vi "界面UI.vi"() -> ()   [LabVIEW 2016, in "德润DR803F超标留样.lvlib"]
uses:
  <vilib>/Utility/miscctls.llb/LVPointTypeDef.ctl
  <vilib>/Utility/config.llb/NI_LVConfig.lvlib
panel:
  in  "超标浓度配置":bool
  out "仪器状态":T1 {"门状态" items=["关闭", "打开"]; "采样模式" items=["定时留样"=1, "时间等比"=2, "同步留样"=3, "外控留样"=4, "超标留样"=5]; "工作进程" items=["清洗管路初始化", "采样瓶位置初始化", "采样瓶排空", "清洗管下降", "采样瓶清洗", "清洗管上升", "外置泵延时", "管路润洗", "进样1", "进样2", "排空管路", "采样瓶位置调整", "待机"]; "仪器时间" format="%<%Y/%m/%d %H:%M:%S>T"; "工作状态" items=["停止", "运行"]}
  in  "采样瓶排空":bool
  out "超标留样等待时间/s":dbl
  in  "流程停止":bool
  in  "流程启动":bool
  out "流程中":bool
  in  "外控留样设置":bool
  in  "外控留样读取":bool
  in  "串口重开":bool
  in  "读取选择":string(combo)
  in  "VISA resource name":refnum<visa-resource-name>="COM10" caption="VISA资源名称"
  in  "写入缓冲区":string
  in  "采样模式":enum16{"定时留样", "时间等比", "同步留样", "外控留样", "超标留样"}(ring)
  in  "采样启动":bool
  in  "切换停止":bool
  in  "切换运行":bool
  in  "时间校准":bool
  out "读取缓冲区":string
  out "source":string
  out "通讯":bool
  # "德润超标留样803F"
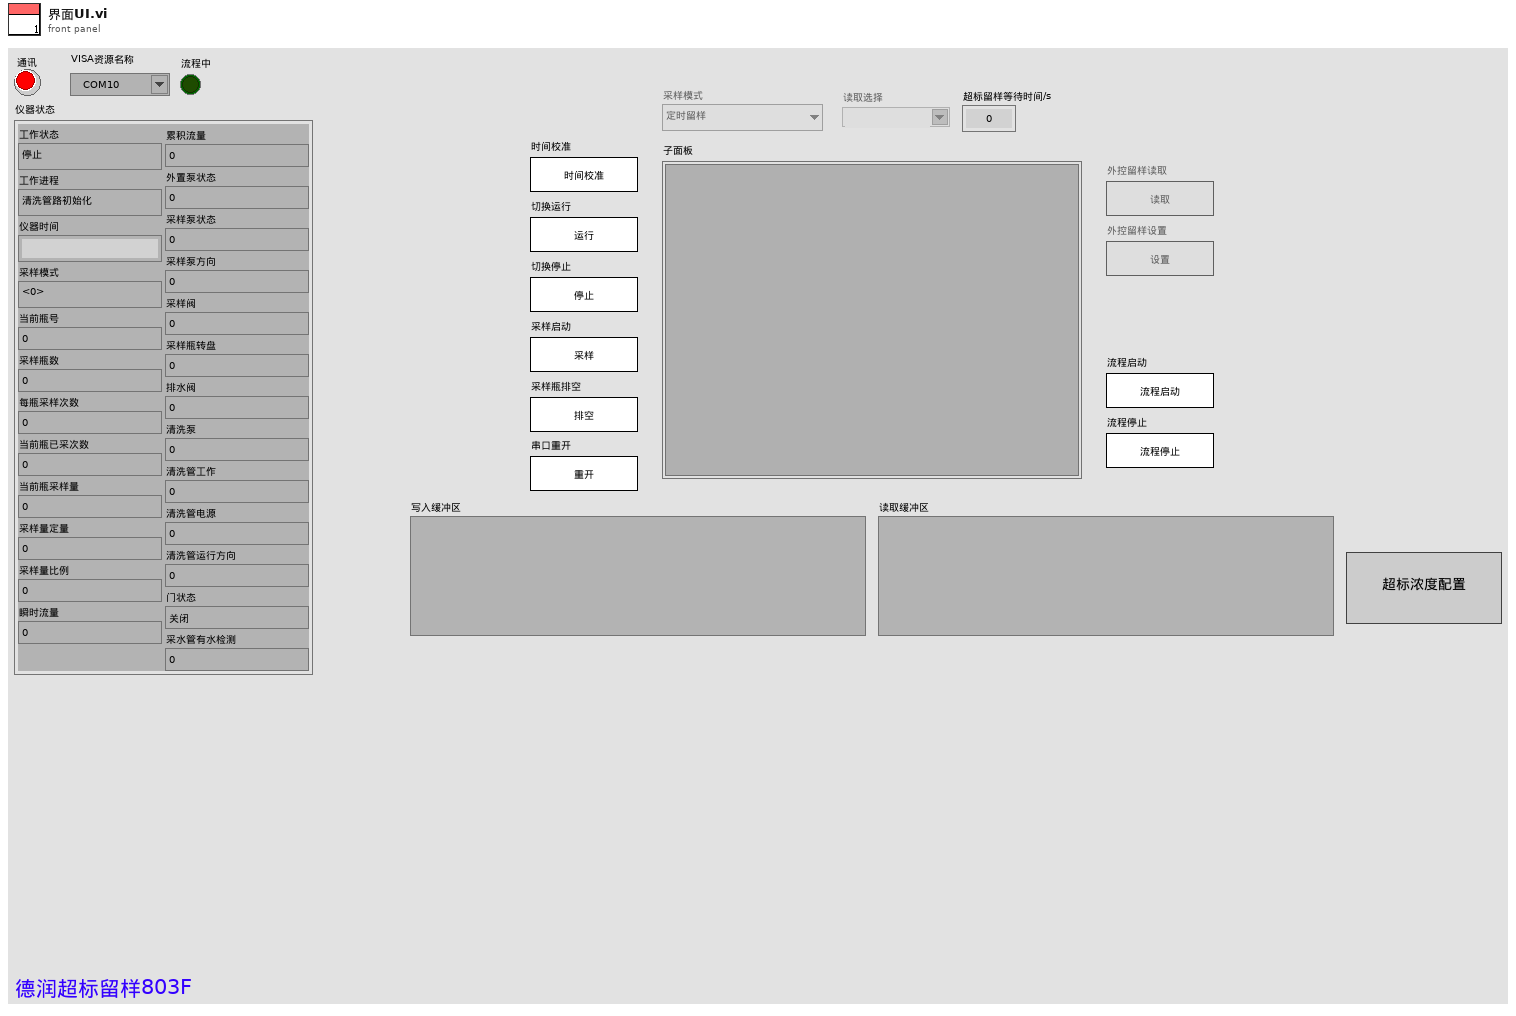
[diagram p1: front panel]
types:
  T1 = cluster{"工作状态":u16, "工作进程":u16, "仪器时间":timestamp, "采样模式":u16, "当前瓶号":dbl, "采样瓶数":dbl, "每瓶采样次数":dbl, "当前瓶已采次数":dbl, "当前瓶采样量":dbl, "采样量定量":dbl, "采样量比例":dbl, "瞬时流量":dbl, "累积流量":dbl, "外置泵状态":dbl, "采样泵状态":dbl, "采样泵方向":dbl, "采样阀":dbl, "采样瓶转盘":dbl, "排水阀":dbl, "清洗泵":dbl, "清洗管工作":dbl, "清洗管电源":dbl, "清洗管运行方向":dbl, "门状态":u16, "采水管有水检测":dbl}
  T2 = cluster{"STEP":enum16{"open", "read", "write", "close"}, "写入缓冲区":string}
  T3 = typedef "LVPointTypeDef.ctl" = cluster{"Horizontal":i16, "Vertical":i16}
  T4 = typedef "NI_LVConfig.lvlib/Config Data RefNum.ctl" = refnum<k1>
  T5 = cluster{"氨氮超标浓度":dbl, "总磷超标浓度":dbl, "总氮超标浓度":dbl, "CODMn超标浓度":dbl, "CODCr超标浓度":dbl}
  T6 = enum32{"Bad", "Idle", "Run top level", "Running"}
  T7 = cluster{"当前瓶号：":dbl, "平行样：":dbl, "留样瓶数：":dbl, "每瓶次数：":dbl, "每次留样：":dbl}
  T8 = cluster{"确定":bool, "氨氮超标浓度":dbl, "总磷超标浓度":dbl, "总氮超标浓度":dbl, "CODMn超标浓度":dbl, "CODCr超标浓度":dbl}
  T9 = enum8{"Enabled", "Disabled", "Disabled and Grayed Out"}
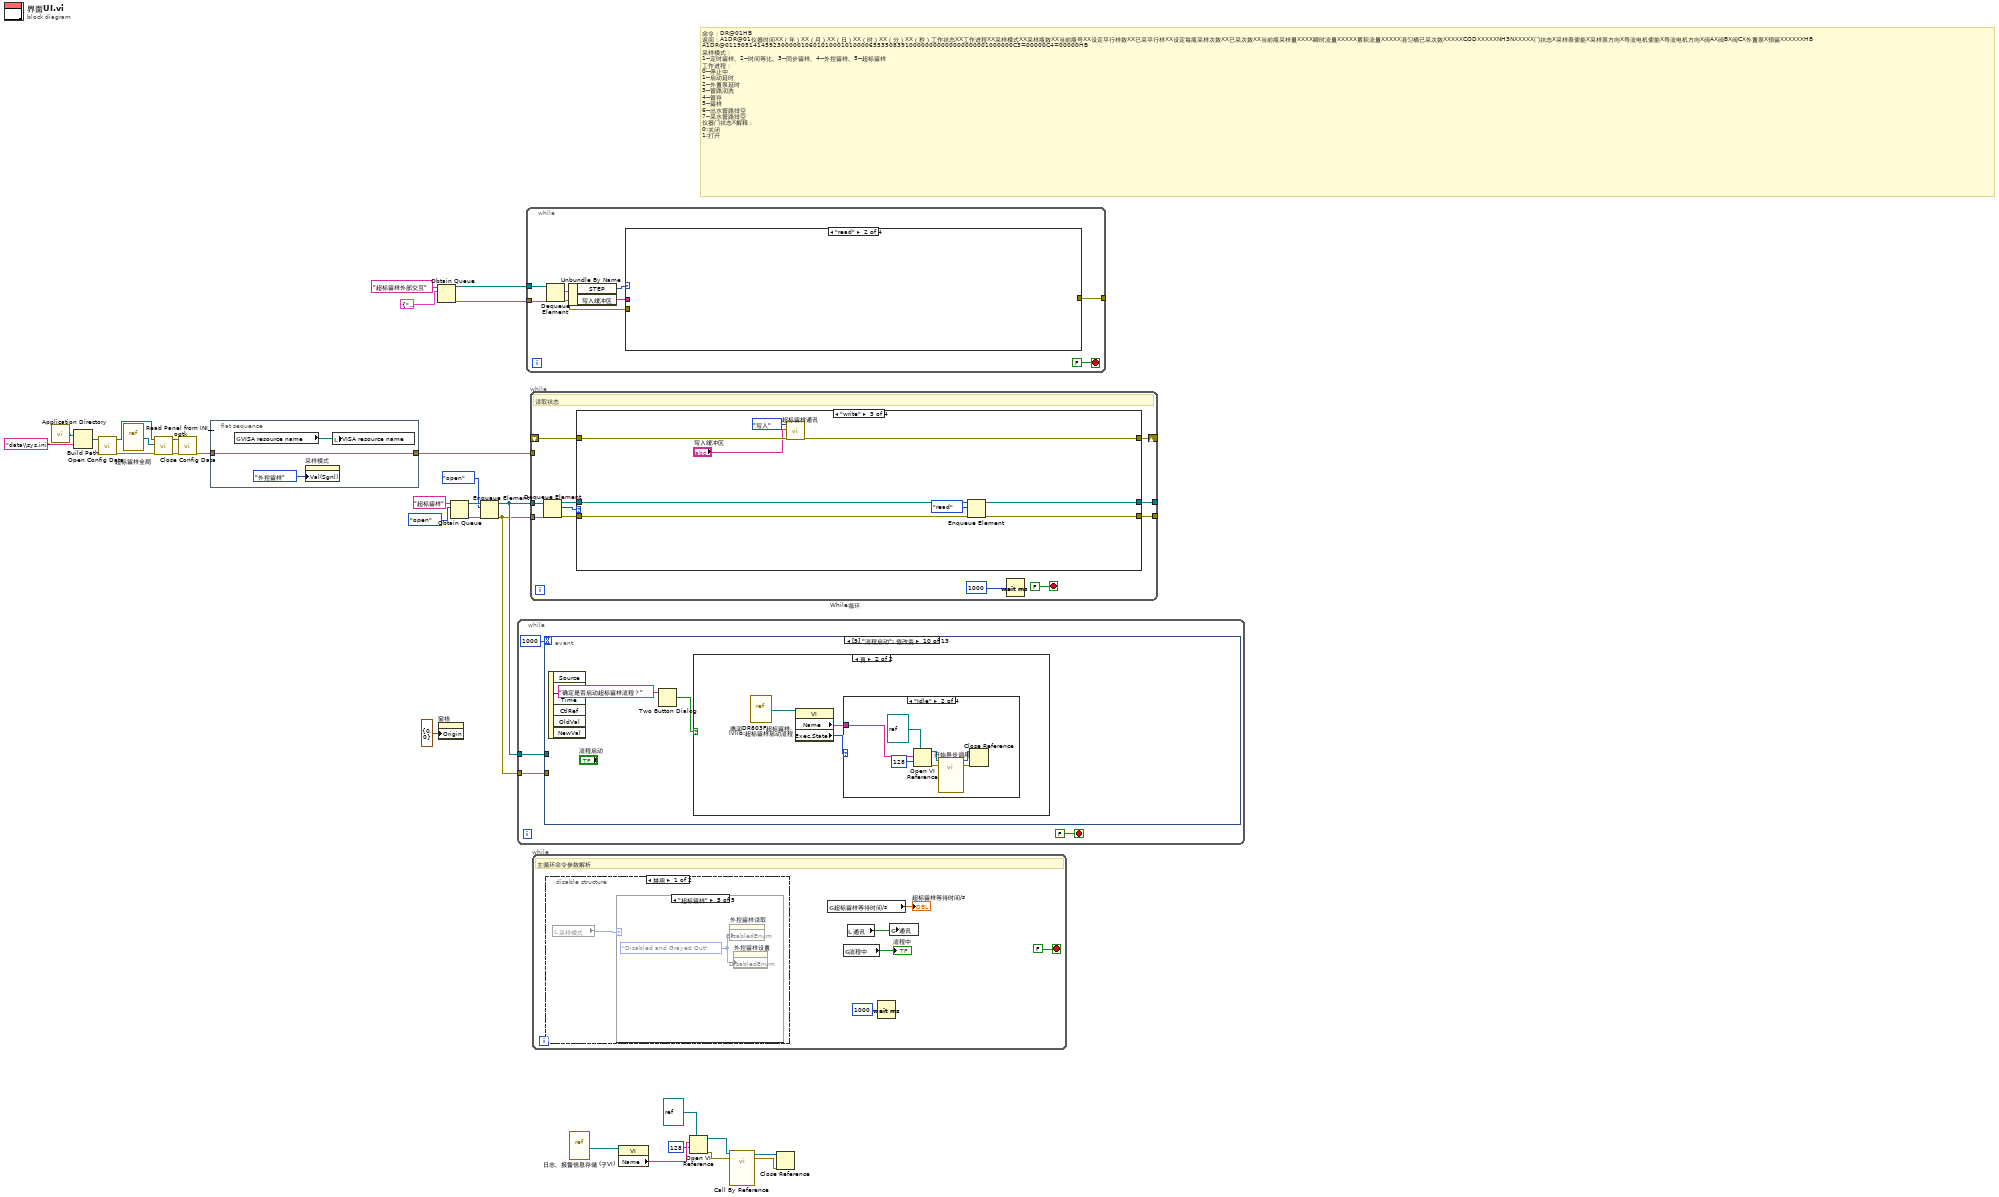
[diagram p0: block diagram]
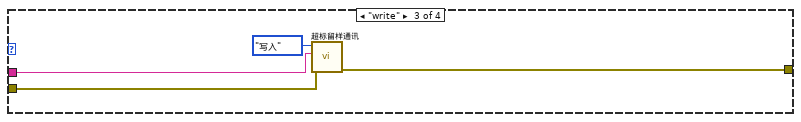
[diagram p3: hidden frame]
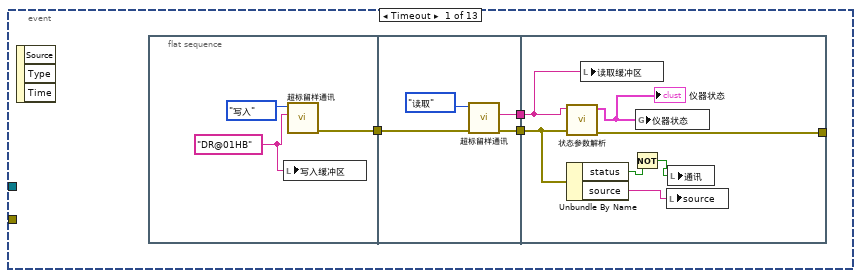
[diagram p5: hidden frame]
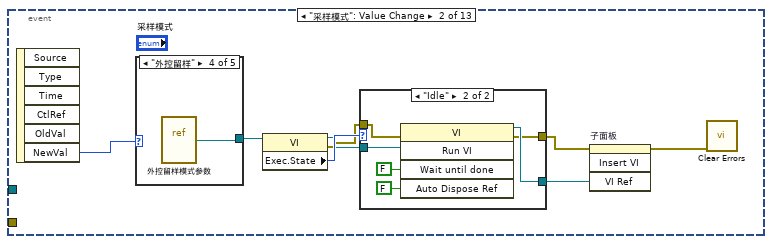
[diagram p6: hidden frame]
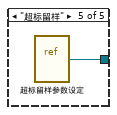
[diagram p11: hidden frame]
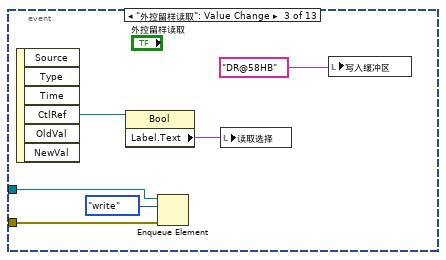
[diagram p12: hidden frame]
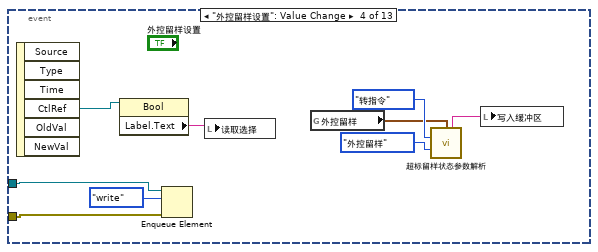
[diagram p13: hidden frame]
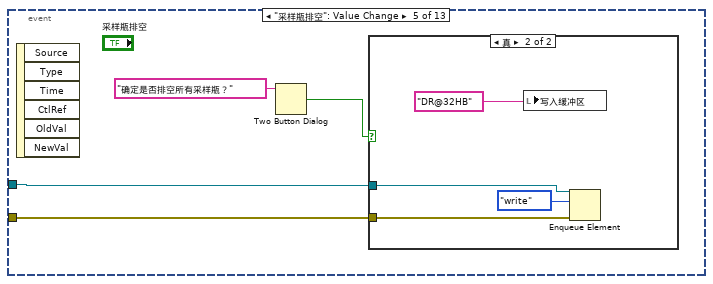
[diagram p14: hidden frame]
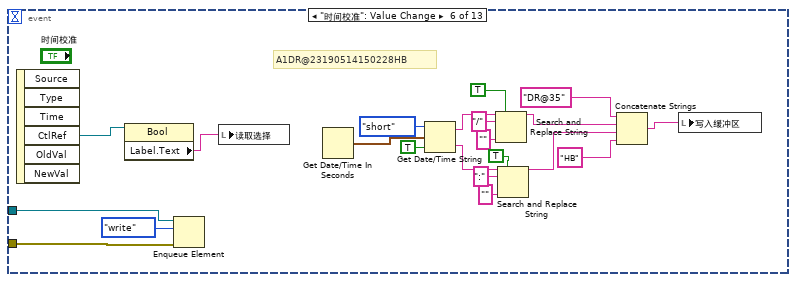
[diagram p16: hidden frame]
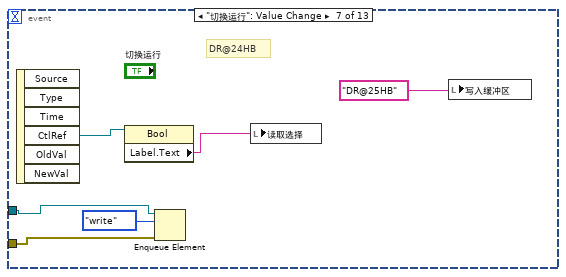
[diagram p17: hidden frame]
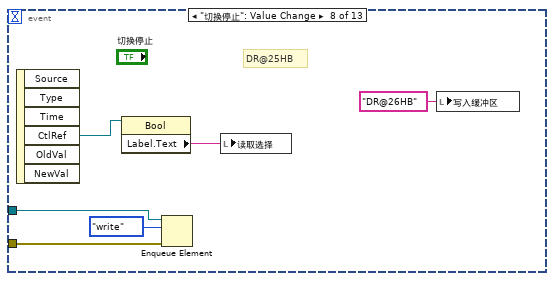
[diagram p18: hidden frame]
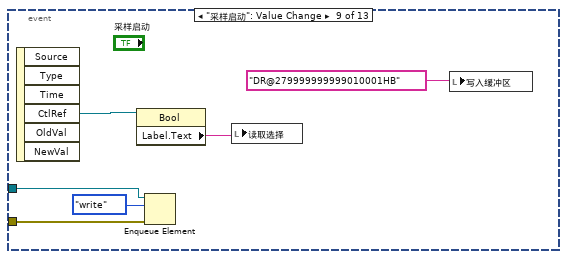
[diagram p19: hidden frame]
diagram:
  # "命令：DR@01HB\n返回：A1DR@01仪器时间XX（年）XX（月）XX（日）XX（时）XX（分）XX（秒）工作状态XX工作进程XX采样模式XX采样瓶数XX当前瓶号XX设定平行样数XX已采平行样XX设定每瓶采样次数XX已采次数XX当前瓶采样量XXXX瞬时流量XXXXX累积流量XXXXX混匀桶已采次数XXXXXCODXXXXXNH3NXXXXX门状态X采样泵使能X采样泵方向X导流电机使能X导流电机方向X阀AX阀BX阀CX外置泵X预留XXXXXXHB\nA1DR@011905141459230000010601010001010000655350839100000000000000000001000000C3=00000C4=00000HB\n采样模式：\n1--定时留样、2--时间等比、3--同步留样、4--外控留样、5--超标留样\n工作进程：\n0--停止中\n1--启动延时\n2--外置泵延时\n3--管路润洗\n4--管存\n5--留样\n6--出水管路排空\n7--采水管路排空\n仪器门状态X解释：\n0:关闭\n1:打开"
  n1 = call <vilib>:"Application Directory.vi"() -> ("Application Directory"=w22:path)
  n2 = Build Path(base path=w22, name or relative path="data\\sys.ini" ("名称或相对路径")) -> (appended path=w20:path)
  n3 = call <vilib>:"Open Config Data.vi"("configuration file path"=w20) -> ("error out"=w16:errorcluster, "refnum"=w19:T4)  [unwired: 8 in, 1 out]
  n4 = vi-ref "超标留样全局.vi"() -> (w18:refnum<vi>)
  n5 = call <userlib>:"Read Panel from INI__ogtk.vi"("error in (no error)"=w16, "VI ref"=w18, "refnum"=w19) -> ("error out"=w15:errorcluster, "refnum out"=w17:T4)  [unwired: 7 in]
  n6 = call <vilib>:"Close Config Data.vi"("error in (no error)"=w15, "refnum"=w17) -> ("error out"=w14:errorcluster)  [unwired: 8 in, 1 out]
  n7 = flat-sequence {
    tunnel: w14 -> [w33]
    tunnel: [w33] -> w13
    frame #0 {
      n8 = global read "超标留样全局.vi" "VISA resource name"() -> (w32:refnum<visa-resource-name>)
      n9 = property on="采样模式" class="Enum (严格)"("Val(Sgnl)"=enum16{"定时留样", "时间等比", "同步留样", "外控留样", "超标留样"}."外控留样" ("采样模式")) -> ()  [unwired: 2 in, 2 out]
      n10 = local write "VISA resource name"(w32) -> ()
    }
  }
  n11 = Obtain Queue(name (unnamed)="超标留样外部交互" ("名称（未命名）"), element data type=T2 {"STEP"=enum."write", "写入缓冲区"="ª\u0006\u0000\u0000P`\u00000»"}) -> (queue out=w11:refnum<queue>, error out=w10:errorcluster)  [unwired: 3 in, 1 out]
  n12 = property on="窗格" class="Pane"("Origin"=T3 {"Horizontal"=0, "Vertical"=0} ("原点")) -> ()  [unwired: 2 in, 2 out]
  n13 = Obtain Queue(name (unnamed)="超标留样" ("名称（未命名）"), element data type=enum16{"open", "read", "write", "close"}."open") -> (queue out=w28:refnum<queue>, error out=w27:errorcluster)  [unwired: 3 in, 1 out]
  n14 = Enqueue Element(queue=w28, element=enum16{"open", "read", "write", "close"}."open", error in (no error)=w27) -> (queue out=w25:refnum<queue>, error out=w24:errorcluster)  [unwired: 1 in, 1 out]
  n15 = while {
    tunnel: w25 -> [w36]
    tunnel: w24 -> [w35]
    stop <- FALSE stop-if-true
    n16 = event shown="[9] \"流程启动\": 值改变" {
      selector: _ -> [_ _ _ _ _ _ _ _ _ _ _ _ _]
      dyn-events: _ -> [_ _ _ _ _ _ _ _ _ _ _ _ _]
      timeout: 1000 -> [_ _ _ _ _ _ _ _ _ _ _ _ _]
      tunnel: w36 -> [_ _ w75 w86 w91 w115 w120 w126 w132 _ w149 w164 _]
      tunnel: w35 -> [_ _ w76 w85 w90 w114 w119 w125 w131 _ w148 w163 _]
      event Timeout {
        n17 = event-data() -> ()  [unwired: 1 in, 3 out]
        n18 = flat-sequence {
          tunnel: [w42] -> w40
          tunnel: w40 -> [w46]
          tunnel: [w45] -> w39
          tunnel: [w44] -> w38
          tunnel: w39 -> [w51]
          tunnel: w38 -> [w53]
          tunnel: [w54] -> _
          frame #0 {
            w41 = "DR@01HB" ("写入缓冲区")
            n19 = local write "写入缓冲区"(w41) -> ()
            n20 = call "超标留样通讯.vi"("写入缓冲区"=w41, "功能输入"=enum16{"打开串口", "写入", "读取", "关闭串口"}."写入") -> ("error out"=w42:errorcluster)  [unwired: 7 in, 2 out]
          }
          frame #1 {
            n21 = call "超标留样通讯.vi"("error in (no error)"=w46, "功能输入"=enum16{"打开串口", "写入", "读取", "关闭串口"}."读取") -> ("error out"=w45:errorcluster, "读取缓冲区"=w44:string)  [unwired: 7 in, 1 out]
          }
          frame #2 {
            n22 = call "状态参数解析.vi"("error in (no error)"=w51, "字符串"=w53) -> ("error out"=w54:errorcluster, "簇"=w52:T1)  [unwired: 8 in]
            "仪器状态" <- w52
            n23 = Unbundle By Name(w51) -> ("status"=w48:bool, "source"=w50:string)
            n24 = local write "读取缓冲区"(w53) -> ()
            n25 = Not(x=w48) -> (.not. x?=w49:bool)
            n26 = global write "超标留样全局.vi" "仪器状态"(w52) -> ()
            n27 = local write "source"(w50) -> ()
            n28 = local write "通讯"(w49) -> ()
          }
        }
      }
      event "采样模式": Value Change {
        n29 = event-data() -> ("NewVal"=w62:enum16{"定时留样", "时间等比", "同步留样", "外控留样", "超标留样"})  [unwired: 1 in, 5 out]
        n30 = case shown="\"外控留样\"" w62 {
          tunnel: [_ _ _ w71 w72] -> w61
          frame "定时留样", Default {
          }
          frame "时间等比" {
          }
          frame "同步留样" {
          }
          frame "外控留样" {
            n31 = vi-ref "外控留样模式参数.vi"() -> (w71:refnum<vi>)
          }
          frame "超标留样" {
            n32 = vi-ref "超标留样参数设定.vi"() -> (w72:refnum<vi>)
          }
        }
        n33 = property class="VI"(reference=w61) -> (reference out=w59:refnum<vi>, error out=w57:errorcluster, "Exec.State"=w60:T6)  [unwired: 1 in]
        n34 = case shown="\"Idle\"" w60 {
          tunnel: w59 -> [w64 w70]
          tunnel: [w64 w67] -> w58
          tunnel: w57 -> [w63 w66]
          tunnel: [w63 w65] -> w56
          frame "Bad", Default {
          }
          frame "Idle" {
            n35 = invoke class="VI" method="Run VI"(reference=w70, error in=w66, "Wait until done"=FALSE ("结束前等待"), "Auto Dispose Ref"=FALSE ("自动销毁引用")) -> (reference out=w67:refnum<vi>, error out=w65:errorcluster)  [unwired: 1 in, 3 out]
          }
        }
        n36 = invoke on="子面板" class="SubPnl" method="Insert VI"(error in=w56, "VI Ref"=w58) -> (error out=w55:errorcluster)  [unwired: 2 in, 3 out]
        n37 = call <vilib>:"Clear Errors.vi"("error in (no error)"=w55) -> ()  [unwired: 5 in, 2 out]
      }
      event "外控留样读取": Value Change {
        n38 = event-data() -> ("CtlRef"=w74:refnum<vi>)  [unwired: 1 in, 5 out]
        n39 = property class="Bool"(reference=w74) -> ("Label.Text"=w73:string)  [unwired: 1 in, 2 out]
        n40 = Enqueue Element(queue=w75, element=enum16{"open", "read", "write", "close"}."write" ("元素"), error in (no error)=w76) -> ()  [unwired: 1 in, 3 out]
        n41 = local write "读取选择"(w73) -> ()
        n42 = local write "写入缓冲区"("DR@58HB") -> ()
      }
      event "外控留样设置": Value Change {
        n43 = event-data() -> ("CtlRef"=w80:refnum<vi>)  [unwired: 1 in, 5 out]
        n44 = property class="Bool"(reference=w80) -> ("Label.Text"=w79:string)  [unwired: 1 in, 2 out]
        n45 = Enqueue Element(queue=w86, element=enum16{"open", "read", "write", "close"}."write" ("元素"), error in (no error)=w85) -> ()  [unwired: 1 in, 3 out]
        n46 = local write "读取选择"(w79) -> ()
        n47 = global read "超标留样全局.vi" "外控留样"() -> (w81:T7)
        n48 = call "超标留样状态参数解析.vi"("外控留样"=w81, "解析/转指令"=enum16{"解析", "转指令"}."转指令", "模式选择"=enum16{"外控留样", "超标留样"}."外控留样") -> ("输出字符串"=w82:string)  [unwired: 11 in, 1 out]
        n49 = local write "写入缓冲区"(w82) -> ()
      }
      event "采样瓶排空": Value Change {
        n50 = event-data() -> ()  [unwired: 1 in, 6 out]
        n51 = Two Button Dialog(message="确定是否排空所有采样瓶？" ("消息")) -> (T button?=w88:bool)  [unwired: 2 in]
        n52 = case shown="真" w88 {
          tunnel: w91 -> [_ w93]
          tunnel: w90 -> [_ w92]
          frame False {
          }
          frame True {
            n53 = local write "写入缓冲区"("DR@32HB") -> ()
            n54 = Enqueue Element(queue=w93, element=enum16{"open", "read", "write", "close"}."write" ("元素"), error in (no error)=w92) -> ()  [unwired: 1 in, 3 out]
          }
        }
      }
      event "时间校准": Value Change {
        # "A1DR@23190514150228HB"
        n55 = event-data() -> ("CtlRef"=w97:refnum<vi>)  [unwired: 1 in, 5 out]
        n56 = property class="Bool"(reference=w97) -> ("Label.Text"=w96:string)  [unwired: 1 in, 2 out]
        n57 = Enqueue Element(queue=w115, element=enum16{"open", "read", "write", "close"}."write" ("元素"), error in (no error)=w114) -> ()  [unwired: 1 in, 3 out]
        n58 = local write "读取选择"(w96) -> ()
        n59 = Get Date/Time In Seconds() -> (seconds since 1Jan1904=w110:timestamp)
        n60 = Get Date/Time String(date format (0)=enum16{"short", "long", "abbreviated"}."short" ("日期格式(0)"), seconds (now)=w110, want seconds? (F)=TRUE ("需要秒？(F)")) -> (date string=w109:string, time string=w102:string)
        n61 = Search and Replace String(replace all?=TRUE ("替换全部？(F)"), input string=w109, search string="/" ("搜索字符串"), replace string="" ("替换字符串(\"\")")) -> (result string=w101:string)  [unwired: 4 in, 3 out]
        n62 = Search and Replace String(replace all?=TRUE ("替换全部？(F)"), input string=w102, search string=":" ("搜索字符串"), replace string="" ("替换字符串(\"\")")) -> (result string=w100:string)  [unwired: 4 in, 3 out]
        n63 = Concatenate Strings("DR@35" ("写入缓冲区"), w101, w100, "HB" ("写入缓冲区")) -> (w98:string)
        n64 = local write "写入缓冲区"(w98) -> ()
      }
      event "切换运行": Value Change {
        # "DR@24HB"
        n65 = event-data() -> ("CtlRef"=w118:refnum<vi>)  [unwired: 1 in, 5 out]
        n66 = property class="Bool"(reference=w118) -> ("Label.Text"=w117:string)  [unwired: 1 in, 2 out]
        n67 = Enqueue Element(queue=w120, element=enum16{"open", "read", "write", "close"}."write" ("元素"), error in (no error)=w119) -> ()  [unwired: 1 in, 3 out]
        n68 = local write "读取选择"(w117) -> ()
        n69 = local write "写入缓冲区"("DR@25HB") -> ()
      }
      event "切换停止": Value Change {
        # "DR@25HB"
        n70 = event-data() -> ("CtlRef"=w124:refnum<vi>)  [unwired: 1 in, 5 out]
        n71 = property class="Bool"(reference=w124) -> ("Label.Text"=w123:string)  [unwired: 1 in, 2 out]
        n72 = Enqueue Element(queue=w126, element=enum16{"open", "read", "write", "close"}."write" ("元素"), error in (no error)=w125) -> ()  [unwired: 1 in, 3 out]
        n73 = local write "读取选择"(w123) -> ()
        n74 = local write "写入缓冲区"("DR@26HB" ("写入缓冲区")) -> ()
      }
      event "采样启动": Value Change {
        n75 = event-data() -> ("CtlRef"=w130:refnum<vi>)  [unwired: 1 in, 5 out]
        n76 = property class="Bool"(reference=w130) -> ("Label.Text"=w129:string)  [unwired: 1 in, 2 out]
        n77 = Enqueue Element(queue=w132, element=enum16{"open", "read", "write", "close"}."write" ("元素"), error in (no error)=w131) -> ()  [unwired: 1 in, 3 out]
        n78 = local write "读取选择"(w129) -> ()
        n79 = local write "写入缓冲区"("DR@279999999999010001HB") -> ()
      }
      event "流程启动": Value Change {
        n80 = event-data() -> ()  [unwired: 1 in, 6 out]
        n81 = Two Button Dialog(message="确定是否启动超标留样流程？" ("消息")) -> (T button?=w135:bool)  [unwired: 2 in]
        n82 = case shown="真" w135 {
          frame False {
          }
          frame True {
            n83 = vi-ref "德润DR803F超标留样.lvlib:超标留样启动流程.vi"() -> (w137:refnum<vi>)
            n84 = property class="VI"(reference=w137) -> ("Name"=w138:string, "Exec.State"=w139:T6)  [unwired: 1 in, 2 out]
            n85 = case shown="\"Idle\"" w139 {
              tunnel: w138 -> [_ w142 _ _]
              frame "Bad", Default {
              }
              frame "Idle" {
                n86 = Open VI Reference(type specifier VI Refnum (for type only)=refnum<vi> refnum ("类型说明符VI引用句柄（仅用于类型）"), vi path=w142, options=128 ("选项")) -> (vi reference=w146:refnum<vi>, error out=w141:errorcluster)  [unwired: 3 in]
                n87 = call-by-ref "开始异步调用"(reference=w146, error in=w141) -> (reference out=w145:refnum<vi>, error out=w140:errorcluster)  [unwired: 12 in]
                n88 = Close Reference(reference=w145, error in (no error)=w140) -> ()  [unwired: 1 out]
              }
              frame "Run top level" {
              }
              frame "Running" {
                n89 = One Button Dialog(message="流程已启动，无需重复启动！" ("消息")) -> ()  [unwired: 1 in, 1 out]
              }
            }
          }
        }
      }
      event "流程停止": Value Change {
        n90 = event-data() -> ()  [unwired: 1 in, 6 out]
        n91 = Two Button Dialog(message="确定是否停止超标留样流程并排空当前瓶？" ("消息")) -> (T button?=w150:bool)  [unwired: 2 in]
        n92 = case shown="真" w150 {
          tunnel: w149 -> [_ w154]
          tunnel: w148 -> [_ w153]
          frame False {
          }
          frame True {
            n93 = Obtain Notifier(name (unnamed)="超标留样流程" ("名称（未命名）"), notification data type=FALSE ("采样完成")) -> (notifier out=w160:refnum<notifier>, error out=w159:errorcluster)  [unwired: 2 in, 1 out]
            n94 = Enqueue Element(queue=w154, element=enum16{"open", "read", "write", "close"}."write" ("元素"), error in (no error)=w153) -> ()  [unwired: 1 in, 3 out]
            n95 = Send Notification(notification=TRUE ("通知"), notifier=w160, error in (no error)=w159) -> (notifier out=w157:refnum<notifier>, error out=w156:errorcluster)
            n96 = Release Notifier(notifier=w157, error in (no error)=w156) -> ()  [unwired: 1 in, 3 out]
            n97 = local write "写入缓冲区"("DR@26HB" ("写入缓冲区")) -> ()
          }
        }
      }
      event "串口重开": Value Change {
        n98 = event-data() -> ()  [unwired: 1 in, 6 out]
        n99 = flat-sequence {
          frame #0 {
            n100 = local read "VISA resource name"() -> (w166:refnum<visa-resource-name>)
            n101 = global write "超标留样全局.vi" "VISA resource name"(w166) -> ()
          }
          frame #1 {
            n102 = call <vilib>:"Application Directory.vi"() -> ("Application Directory"=w168:path)
            n103 = Build Path(base path=w168, name or relative path="data\\sys.ini" ("名称或相对路径")) -> (appended path=w169:path)
            n104 = call <vilib>:"Open Config Data.vi"("configuration file path"=w169) -> ("error out"=w173:errorcluster, "refnum"=w170:T4)  [unwired: 8 in, 1 out]
            n105 = vi-ref "超标留样全局.vi"() -> (w171:refnum<vi>)
            n106 = call <userlib>:"Write Panel to INI__ogtk.vi"("error in (no error)"=w173, "VI ref"=w171, "refnum"=w170) -> ("error out"=w174:errorcluster, "refnum out"=w172:T4)  [unwired: 7 in]
            n107 = call <vilib>:"Close Config Data.vi"("error in (no error)"=w174, "refnum"=w172) -> ("error out"=w179:errorcluster, "file path"=w180:path)  [unwired: 8 in]
            n108 = Open/Create/Replace File(file path (use dialog)=w180, error in=w179) -> (refnum out=w176:refnum<file>, error out=w175:errorcluster)  [unwired: 4 in, 1 out]
            n109 = Flush File(refnum=w176, error in=w175) -> (refnum out=w177:refnum<file>, error out=w178:errorcluster)
            n110 = Close File(refnum=w177, error in=w178) -> ()  [unwired: 2 out]
          }
        }
        n111 = Enqueue Element(queue=w164, element=enum16{"open", "read", "write", "close"}."close" ("元素"), error in (no error)=w163) -> ()  [unwired: 1 in, 3 out]
      }
      event "超标浓度配置": Value Change {
        n112 = event-data() -> ()  [unwired: 1 in, 6 out]
        n113 = global read "超标留样全局.vi" "CODMn超标浓度"() -> (w192:dbl)
        n114 = global read "超标留样全局.vi" "CODCr超标浓度"() -> (w193:dbl)
        n115 = global read "超标留样全局.vi" "总氮超标浓度"() -> (w191:dbl)
        n116 = global read "超标留样全局.vi" "总磷超标浓度"() -> (w190:dbl)
        n117 = global read "超标留样全局.vi" "氨氮超标浓度"() -> (w189:dbl)
        n118 = Bundle By Name(cluster=T5 {"氨氮超标浓度"=0.0, "总磷超标浓度"=0.0, "总氮超标浓度"=0.0, "CODMn超标浓度"=0.0, "CODCr超标浓度"=0.0} ("输入"), "氨氮超标浓度"=w189, "总磷超标浓度"=w190, "总氮超标浓度"=w191, "CODMn超标浓度"=w192, "CODCr超标浓度"=w193) -> (w188:T5)
        n119 = call "超标浓度设置.vi"("输入"=w188) -> ("输出"=w187:T8)  [unwired: 10 in]
        n120 = Unbundle By Name(w187) -> ("确定"=w186:bool, "氨氮超标浓度"=w181:dbl, "总磷超标浓度"=w182:dbl, "总氮超标浓度"=w183:dbl, "CODMn超标浓度"=w184:dbl, "CODCr超标浓度"=w185:dbl)
        n121 = case shown="真" w186 {
          tunnel: w185 -> [_ w199]
          tunnel: w184 -> [_ w198]
          tunnel: w183 -> [_ w197]
          tunnel: w182 -> [_ w196]
          tunnel: w181 -> [_ w195]
          frame False {
          }
          frame True {
            n122 = flat-sequence {
              tunnel: w199 -> [w204]
              tunnel: w198 -> [w203]
              tunnel: w197 -> [w202]
              tunnel: w196 -> [w201]
              tunnel: w195 -> [w200]
              frame #0 {
                n123 = global write "超标留样全局.vi" "CODMn超标浓度"(w203) -> ()
                n124 = global write "超标留样全局.vi" "CODCr超标浓度"(w204) -> ()
                n125 = global write "超标留样全局.vi" "总氮超标浓度"(w202) -> ()
                n126 = global write "超标留样全局.vi" "总磷超标浓度"(w201) -> ()
                n127 = global write "超标留样全局.vi" "氨氮超标浓度"(w200) -> ()
              }
              frame #1 {
                n128 = call <vilib>:"Application Directory.vi"() -> ("Application Directory"=w206:path)
                n129 = Build Path(base path=w206, name or relative path="data\\sys.ini" ("名称或相对路径")) -> (appended path=w207:path)
                n130 = call <vilib>:"Open Config Data.vi"("configuration file path"=w207) -> ("error out"=w211:errorcluster, "refnum"=w208:T4)  [unwired: 8 in, 1 out]
                n131 = vi-ref "超标留样全局.vi"() -> (w209:refnum<vi>)
                n132 = call <userlib>:"Write Panel to INI__ogtk.vi"("error in (no error)"=w211, "VI ref"=w209, "refnum"=w208) -> ("error out"=w212:errorcluster, "refnum out"=w210:T4)  [unwired: 7 in]
                n133 = call <vilib>:"Close Config Data.vi"("error in (no error)"=w212, "refnum"=w210) -> ("error out"=w217:errorcluster, "file path"=w218:path)  [unwired: 8 in]
                n134 = Open/Create/Replace File(file path (use dialog)=w218, error in=w217) -> (refnum out=w214:refnum<file>, error out=w213:errorcluster)  [unwired: 4 in, 1 out]
                n135 = Flush File(refnum=w214, error in=w213) -> (refnum out=w215:refnum<file>, error out=w216:errorcluster)
                n136 = Close File(refnum=w215, error in=w216) -> ()  [unwired: 2 out]
              }
            }
          }
        }
      }
    }
  }
  n137 = while {
    tunnel: w11 -> [w226]
    tunnel: w10 -> [w225]
    tunnel: [w219] -> _
    stop <- FALSE stop-if-true
    n138 = Dequeue Element(queue=w226, error in (no error)=w225) -> (element=w223:T2, error out=w220:errorcluster)  [unwired: 1 in, 2 out]
    n139 = Unbundle By Name(w223) -> ("STEP"=w222:enum16{"open", "read", "write", "close"}, "写入缓冲区"=w221:string)
    n140 = case shown="\"read\"" w222 {
      tunnel: w221 -> [_ _ w230 _]
      tunnel: w220 -> [_ _ w228 _]
      tunnel: [_ _ w227 _] -> w219
      frame "open", Default {
      }
      frame "read" {
      }
      frame "write" {
        n141 = call "超标留样通讯.vi"("error in (no error)"=w228, "写入缓冲区"=w230, "功能输入"=enum16{"打开串口", "写入", "读取", "关闭串口"}."写入") -> ("error out"=w227:errorcluster)  [unwired: 6 in, 2 out]
      }
      frame "close" {
      }
    }
  }
  n142 = while "While循环" {
    tunnel: w25 -> [w239]
    tunnel: w24 -> [w238]
    tunnel: [w234] -> _
    tunnel: [w233] -> _
    shift-right: [w231] -> _
    shift-left: _ -> [w232]
    tunnel: w13 -> [_]
    stop <- FALSE stop-if-true
    # "读取状态"
    n143 = Dequeue Element(queue=w239, error in (no error)=w238) -> (queue out=w236:refnum<queue>, element=w237:enum16{"open", "read", "write", "close"}, error out=w235:errorcluster)  [unwired: 1 in, 1 out]
    n144 = case shown="\"write\"" w237 {
      tunnel: [w245 w247 w279 w291] -> w231
      tunnel: w236 -> [w244 w254 w284 w290]
      tunnel: w235 -> [w243 w253 w283 w289]
      tunnel: [w244 w254 w282 w287] -> w234
      tunnel: [w243 w253 w281 w286] -> w233
      tunnel: w232 -> [_ w256 w280 w293]
      frame "open", Default {
        (unwired) refnum<visa-resource-name> "COM2" ("VISA resource name")
        n145 = global write "超标留样全局.vi" "VISA resource name"("VISA resource name") -> ()
        n146 = call "超标留样通讯.vi"("VISA resource name"="VISA resource name", "功能输入"=enum16{"打开串口", "写入", "读取", "关闭串口"}."打开串口") -> ("error out"=w245:errorcluster)  [unwired: 7 in, 2 out]
      }
      frame "read" {
        n147 = call "超标留样通讯.vi"("error in (no error)"=w256, "功能输入"=enum16{"打开串口", "写入", "读取", "关闭串口"}."读取") -> ("error out"=w247:errorcluster, "读取缓冲区"=w251:string)  [unwired: 7 in, 1 out]
        "读取缓冲区" <- w251
        n148 = case shown="\"外控留样读取\"" "读取选择" {
          tunnel: w251 -> [w257 w264 w271]
          frame "超标留样读取" {
            n149 = flat-sequence {
              tunnel: w257 -> [w260]
              frame #0 {
                n150 = call "超标留样状态参数解析.vi"("输入字符串"=w260, "解析/转指令"=enum16{"解析", "转指令"}."解析", "模式选择"=enum16{"外控留样", "超标留样"}."超标留样") -> ()  [unwired: 11 in, 2 out]
              }
              frame #1 {
                n151 = global write "超标留样全局.vi" "读取更新"(TRUE ("读取更新")) -> ()
              }
              frame #2 {
                n152 = Wait (ms)(milliseconds to wait=u32 500 ("等待时间（毫秒）")) -> ()  [unwired: 1 out]
              }
              frame #3 {
                n153 = global write "超标留样全局.vi" "读取更新"(FALSE ("读取更新")) -> ()
              }
            }
          }
          frame "外控留样读取" {
            n154 = flat-sequence {
              tunnel: w264 -> [w265]
              frame #0 {
                n155 = call "超标留样状态参数解析.vi"("输入字符串"=w265, "解析/转指令"=enum16{"解析", "转指令"}."解析", "模式选择"=enum16{"外控留样", "超标留样"}."外控留样") -> ()  [unwired: 11 in, 2 out]
              }
              frame #1 {
                n156 = global write "超标留样全局.vi" "外控留样读取更新"(TRUE ("读取更新")) -> ()
              }
              frame #2 {
                n157 = Wait (ms)(milliseconds to wait=u32 500 ("等待时间（毫秒）")) -> ()  [unwired: 1 out]
              }
              frame #3 {
                n158 = global write "超标留样全局.vi" "外控留样读取更新"(FALSE ("读取更新")) -> ()
              }
            }
          }
          frame "超标留样设置", Default {
            n159 = disable-structure shown="禁用" {
              disable-tunnel: w271 -> [w276 _]
              frame Disabled {
                n160 = String Subset(string=w276, offset (0)=5 ("偏移量(0)")) -> (substring=w274:string)  [unwired: 1 in]
                n161 = Search/Split String(string=w274, search string/char (-)="HB" ("搜索字符串/字符(-)")) -> (substring before match=w272:string)  [unwired: 1 in, 2 out]
                n162 = One Button Dialog(message=w272) -> ()  [unwired: 1 in, 1 out]
              }
              frame Enabled {
              }
            }
          }
        }
        n163 = Unbundle By Name(w247) -> ("status"=w248:bool, "source"=→"source":string)
        n164 = Not(x=w248) -> (.not. x?=→"通讯":bool)
      }
      frame "write" {
        n165 = call "超标留样通讯.vi"("error in (no error)"=w280, "写入缓冲区"="写入缓冲区", "功能输入"=enum16{"打开串口", "写入", "读取", "关闭串口"}."写入") -> ("error out"=w279:errorcluster)  [unwired: 6 in, 2 out]
        n166 = Enqueue Element(queue=w284, element=enum16{"open", "read", "write", "close"}."read" ("元素"), error in (no error)=w283) -> (queue out=w282:refnum<queue>, error out=w281:errorcluster)  [unwired: 1 in, 1 out]
      }
      frame "close" {
        n167 = call "超标留样通讯.vi"("error in (no error)"=w293, "功能输入"=enum16{"打开串口", "写入", "读取", "关闭串口"}."关闭串口") -> ("error out"=w291:errorcluster)  [unwired: 7 in, 2 out]
        n168 = Enqueue Element(queue=w290, element=enum16{"open", "read", "write", "close"}."open" ("元素"), error in (no error)=w289) -> (queue out=w287:refnum<queue>, error out=w286:errorcluster)  [unwired: 1 in, 1 out]
      }
    }
    n169 = Wait (ms)(milliseconds to wait=u32 1000 ("等待时间（毫秒）")) -> ()  [unwired: 1 out]
  }
  n170 = while {
    stop <- FALSE stop-if-true
    # "主循环命令参数解析"
    n171 = disable-structure shown="禁用" {
      frame Disabled {
        n172 = local read "采样模式"() -> (w299:enum16{"定时留样", "时间等比", "同步留样", "外控留样", "超标留样"})
        n173 = case shown="\"超标留样\"" w299 {
          frame "定时留样", Default {
            w300 = T9."Disabled and Grayed Out" ("禁用")
            n174 = property on="外控留样读取" class="Bool"("DisabledEnum"=w300) -> ()  [unwired: 2 in, 2 out]
            n175 = property on="外控留样设置" class="Bool"("DisabledEnum"=w300) -> ()  [unwired: 2 in, 2 out]
          }
          frame "时间等比" {
          }
          frame "同步留样" {
          }
          frame "外控留样" {
            w301 = T9."Enabled" ("禁用")
            n176 = property on="外控留样读取" class="Bool"("DisabledEnum"=w301) -> ()  [unwired: 2 in, 2 out]
            n177 = property on="外控留样设置" class="Bool"("DisabledEnum"=w301) -> ()  [unwired: 2 in, 2 out]
          }
          frame "超标留样" {
            w302 = T9."Disabled and Grayed Out" ("禁用")
            n178 = property on="外控留样读取" class="Bool"("DisabledEnum"=w302) -> ()  [unwired: 2 in, 2 out]
            n179 = property on="外控留样设置" class="Bool"("DisabledEnum"=w302) -> ()  [unwired: 2 in, 2 out]
          }
        }
      }
      frame Enabled {
      }
    }
    n180 = global read "超标留样全局.vi" "超标留样等待时间/s"() -> (→"超标留样等待时间/s":dbl)
    n181 = global read "超标留样全局.vi" "流程中"() -> (→"流程中":bool)
    n182 = local read "通讯"() -> (w296:bool)
    n183 = Wait (ms)(milliseconds to wait=u32 1000 ("等待时间（毫秒）")) -> ()  [unwired: 1 out]
    n184 = global write "超标留样全局.vi" "通讯"(w296) -> ()
  }
  n185 = vi-ref "日志、报警信息存储 (子VI).vi"() -> (w8:refnum<vi>)
  n186 = property class="VI"(reference=w8) -> ("Name"=w7:string)  [unwired: 1 in, 2 out]
  n187 = Open VI Reference(type specifier VI Refnum (for type only)=refnum<vi> refnum ("类型说明符VI引用句柄（仅用于类型）"), vi path=w7, options=128 ("选项")) -> (vi reference=w5:refnum<vi>, error out=w3:errorcluster)  [unwired: 3 in]
  n188 = call-by-ref "?"(reference=w5, error in=w3) -> (reference out=w2:refnum<vi>, error out=w1:errorcluster)  [unwired: 12 in]
  n189 = Close Reference(reference=w2, error in (no error)=w1) -> ()  [unwired: 1 out]
